vi "Morph_Poly.vi"   [LabVIEW 2022 SP3]
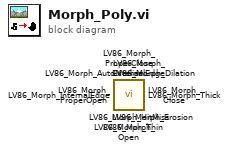
[diagram p0: block diagram]
diagram:
  n1 = call <vilib>:"LV86_Morph_HitMiss.vi"() -> ()  [unwired: 3 in, 1 out]
  n2 = call <vilib>:"LV86_Morph_ExternalEdge.vi"() -> ()  [unwired: 3 in, 1 out]
  n3 = call <vilib>:"LV86_Morph_InternalEdge.vi"() -> ()  [unwired: 3 in, 1 out]
  n4 = call <vilib>:"LV86_Morph_Thick.vi"() -> ()  [unwired: 3 in, 1 out]
  n5 = call <vilib>:"LV86_Morph_Thin.vi"() -> ()  [unwired: 3 in, 1 out]
  n6 = call <vilib>:"LV86_Morph_AutoMedian.vi"() -> ()  [unwired: 3 in, 1 out]
  n7 = call <vilib>:"LV86_Morph_ProperClose.vi"() -> ()  [unwired: 3 in, 1 out]
  n8 = call <vilib>:"LV86_Morph_ProperOpen.vi"() -> ()  [unwired: 3 in, 1 out]
  n9 = call <vilib>:"LV86_Morph_Close.vi"() -> ()  [unwired: 3 in, 1 out]
  n10 = call <vilib>:"LV86_Morph_Open.vi"() -> ()  [unwired: 3 in, 1 out]
  n11 = call <vilib>:"LV86_Morph_Erosion.vi"() -> ()  [unwired: 3 in, 1 out]
  n12 = call <vilib>:"LV86_Morph_Dilation.vi"() -> ()  [unwired: 3 in, 1 out]
